vi "Write Channels.vi"(8 "error in (no error)":errorcluster, 10 "Channels":cluster{"Count":u16, "Channel":T1[]}, 11 "FgenPluginsBase in":refnum<class "FgenPluginsBase.lvclass">) -> (0 "error out":errorcluster, 3 "FgenPluginsBase out":refnum<class "FgenPluginsBase.lvclass">)   [LabVIEW 2018, in "FgenPlugins.lvlib" / "FgenPluginsBase.lvclass"]
uses:
  FgenPluginsBase.lvclass
  TypeDefs/Channel.ctl
  FgenPluginsBase.lvclass/FgenPluginsBase.ctl
  FgenPlugins.lvlib
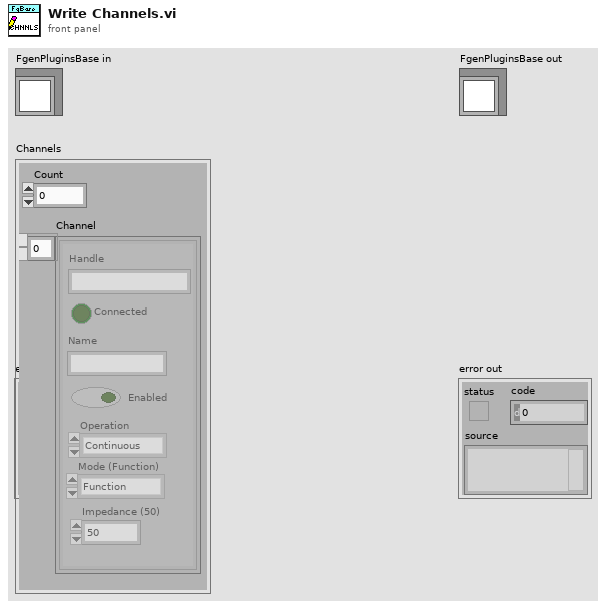
[diagram p1: front panel]
types:
  T1 = typedef "FgenPlugins.lvlib/Channel.ctl" = cluster{"Name":string, "Enabled":bool, "Operation":enum16{"Continuous", "Burst"}, "Impedance (50)":dbl, "Handle":string, "Connected":bool, "Mode (Function)":enum16{"Function", "Arbitrary", "Sequence"}}
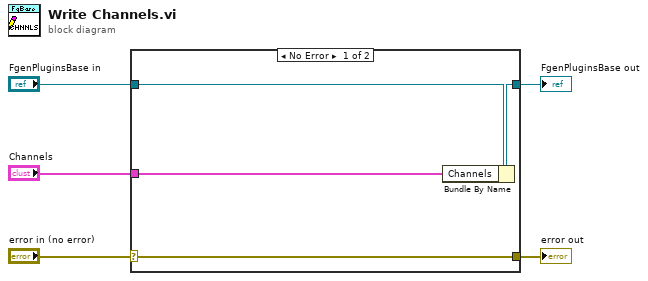
[diagram p0: block diagram]
diagram:
  n1 = case shown="No Error" "error in (no error)" {
    selector: "error in (no error)" -> [w9 w10]
    tunnel: [w9 w10] -> w4
    tunnel: [w7 w11] -> w2
    tunnel: "FgenPluginsBase in" -> [w8 w11]
    tunnel: "Channels" -> [w6 _]
    frame No Error {
      n2 = Bundle By Name(cluster=w8, "Channels"=w6) -> (w7:refnum<class "FgenPluginsBase.lvclass">)
    }
    frame Error {
    }
  }
  "error out" <- w4
  "FgenPluginsBase out" <- w2
